vi "condAmbientalesFinales.vi"(8 "error in (no error)":errorcluster, 11 "Sonometro in":refnum<class "Sonometro.lvclass">) -> (0 "error out":errorcluster, 3 "Sonometro out":refnum<class "Sonometro.lvclass">)   [LabVIEW 2019, in "Sonometro.lvclass"]
uses:
  Sonometro.lvclass
  Base de Datos/Base de Datos.lvclass
  Base de Datos/SQLiteConnector/SQLiteConnection.lvclass
panel:
  in  "salir":bool
  in  "presion":dbl
  out "presion_corregida":dbl
  out "presion_ok":bool
  in  "humedad":dbl
  out "humedad_corregida":dbl
  out "humedad_ok":bool
  in  "temperatura":dbl
  out "temp_corregida":dbl
  out "temp_ok":bool
  # "Medido"
  # "Corregido"
  # "Cumple"
  # "Humedad [%]"
  # "Presión [hPa]"
  # "Temperatura [°C]"
  # "Condiciones Ambientales \nFINALES"
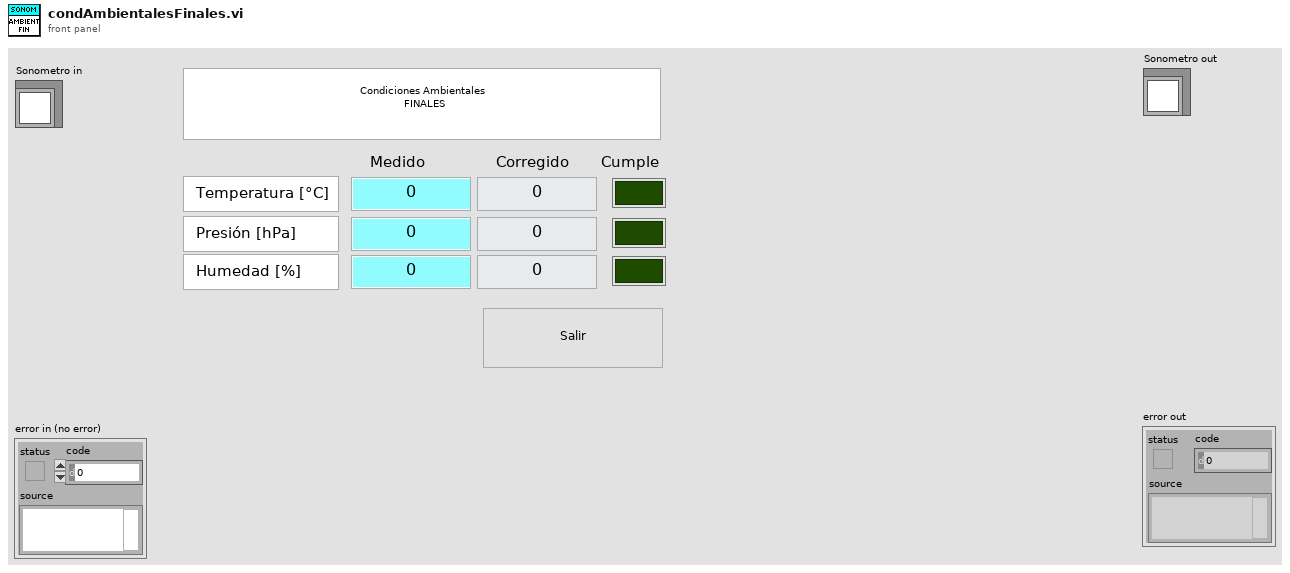
[diagram p1: front panel]
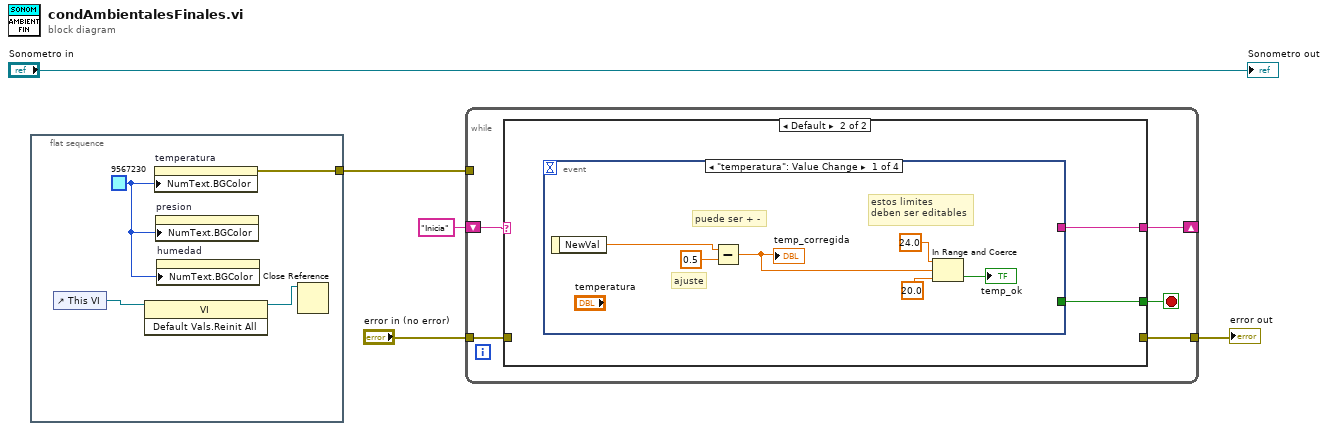
[diagram p0: block diagram]
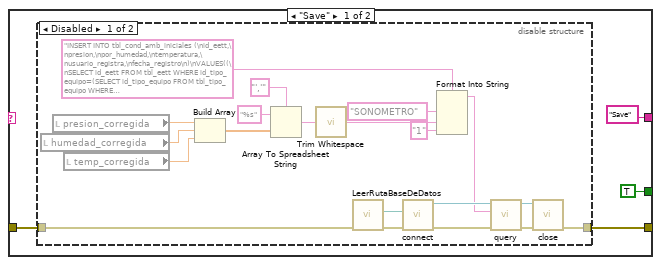
[diagram p2: hidden frame]
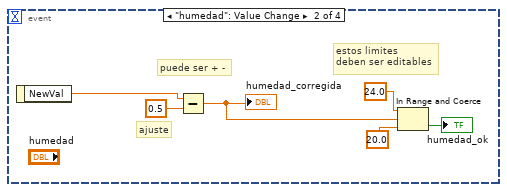
[diagram p4: hidden frame]
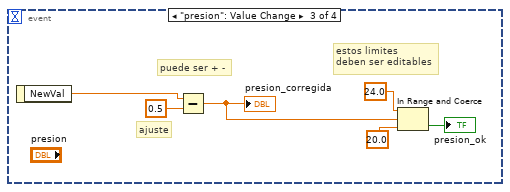
[diagram p5: hidden frame]
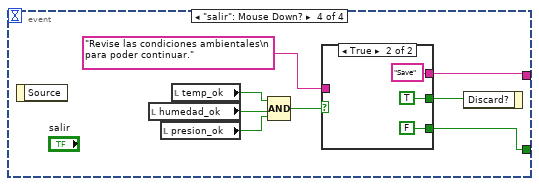
[diagram p6: hidden frame]
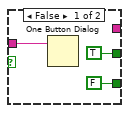
[diagram p7: hidden frame]
diagram:
  n1 = flat-sequence {
    tunnel: [w8] -> w4
    frame #0 {
      w9 = u32 9567230
      n2 = control-ref of="This VI"() -> (w7:refnum<vi>)
      n3 = invoke class="VI" method="Default Vals.Reinit All"(reference=w7) -> (reference out=w6:refnum<vi>)  [unwired: 2 in, 2 out]
      n4 = property on="temperatura" class="DigNum (strict)"("NumText.BGColor"=w9) -> (error out=w8:errorcluster)  [unwired: 2 in, 1 out]
      n5 = property on="presion" class="DigNum (strict)"("NumText.BGColor"=w9) -> ()  [unwired: 2 in, 2 out]
      n6 = property on="humedad" class="DigNum (strict)"("NumText.BGColor"=w9) -> ()  [unwired: 2 in, 2 out]
      n7 = Close Reference(reference=w6) -> ()  [unwired: 1 in, 1 out]
    }
  }
  n8 = while {
    tunnel: w4 -> [_]
    shift-right: [w12] -> _
    shift-left: "Inicia" -> [w13]
    tunnel: [w11] -> w1
    tunnel: "error in (no error)" -> [w10]
    stop <- w14 stop-if-true
    n9 = case shown="Default" w13 {
      tunnel: [TRUE w41] -> w14
      tunnel: ["Save" w40] -> w12
      tunnel: [w16 _] -> w11
      tunnel: w10 -> [w15 _]
      frame "Save" {
        n10 = disable-structure shown="Disabled" {
          disable-tunnel: [w20 w39] -> w16
          disable-tunnel: w15 -> [w19 w39]
          frame Disabled {
            n11 = local read "humedad_corregida"() -> (w29:dbl)
            n12 = local read "presion_corregida"() -> (w28:dbl)
            n13 = local read "temp_corregida"() -> (w30:dbl)
            n14 = Build Array(w28, w29, w30) -> (w27:dbl[])
            n15 = Array To Spreadsheet String(delimiter (Tab)="','", array=w27, 3:"%s" ("format string")) -> (spreadsheet string=w23:string)
            n16 = call <vilib>:"Trim Whitespace.vi"("string"=w23) -> ("trimmed string"=w22:string)  [unwired: 1 in]
            n17 = call "LeerRutaBaseDeDatos.vi"("error in (no error)"=w19) -> ("error out"=w33:errorcluster, "Database Path"=w34:path)  [unwired: 9 in]
            n18 = call "connect.vi"("error in (no error)"=w33, "Database Path"=w34) -> ("error out"=w36:errorcluster, "object out"=w35:refnum<class "SQLiteConnection.lvclass">)  [unwired: 8 in]
            n19 = Format Into String(format string="INSERT INTO tbl_cond_amb_iniciales (\nid_eett,\npresion,\npor_humedad,\ntemperatura,\nusuario_registra,\nfecha_registro\n)\nVALUES((\nSELECT id_eett FROM tbl_eett WHERE id_tipo_equipo=(SELECT id_tipo_equipo FROM tbl_tipo_equipo WHERE nombre='%s')),'%s','%s',DATETIME('NOW'))" ("SQL Statement"), "SONOMETRO" ("input 1"), w22, "1" ("input 2")) -> (resulting string=w31:string)  [unwired: 2 in, 1 out]
            n20 = call "query.vi"("error in (no error)"=w36, "SQL Statement"=w31, "object in"=w35) -> ("error out"=w38:errorcluster, "object out"=w37:refnum<class "SQLiteConnection.lvclass">)  [unwired: 5 in, 2 out]
            n21 = call-dynamic "close.vi"("error in (no error)"=w38, "object in"=w37) -> ("error out"=w20:errorcluster)  [unwired: 8 in, 1 out]
          }
          frame Enabled {
            # "Cambiar a codigo para BD de condiciones ambientales finales en Sonometro"
          }
        }
      }
      frame Default {
        n22 = event shown="[0] \"temperatura\": Value Change" {
          selector: _ -> [_ _ _ _]
          dyn-events: _ -> [_ _ _ _]
          timeout: _ -> [_ _ _ _]
          tunnel: [_ _ _ w61] -> w41
          tunnel: [_ _ _ w60] -> w40
          event "temperatura": Value Change {
            # "estos limites\ndeben ser editables"
            # "puede ser + -"
            # "ajuste"
            n23 = event-data() -> ("NewVal"=w42:dbl)  [unwired: 1 in]
            n24 = Subtract(x=w42, y=0.5) -> (x-y=w47:dbl)
            "temp_corregida" <- w47
            n25 = In Range and Coerce(upper limit=24.0, x=w47, lower limit=20.0) -> (In Range?=→"temp_ok":bool)  [unwired: 1 out]
          }
          event "humedad": Value Change {
            # "estos limites\ndeben ser editables"
            # "puede ser + -"
            # "ajuste"
            n26 = event-data() -> ("NewVal"=w50:dbl)  [unwired: 1 in]
            n27 = Subtract(x=w50, y=0.5) -> (x-y=w49:dbl)
            "humedad_corregida" <- w49
            n28 = In Range and Coerce(upper limit=24.0, x=w49, lower limit=20.0) -> (In Range?=→"humedad_ok":bool)  [unwired: 1 out]
          }
          event "presion": Value Change {
            # "estos limites\ndeben ser editables"
            # "puede ser + -"
            # "ajuste"
            n29 = event-data() -> ("NewVal"=w56:dbl)  [unwired: 1 in]
            n30 = Subtract(x=w56, y=0.5) -> (x-y=w55:dbl)
            "presion_corregida" <- w55
            n31 = In Range and Coerce(upper limit=24.0, x=w55, lower limit=20.0) -> (In Range?=→"presion_ok":bool)  [unwired: 1 out]
          }
          event "salir": Mouse Down? {
            n32 = event-data() -> ()  [unwired: 1 in, 1 out]
            n33 = local read "humedad_ok"() -> (w66:bool)
            n34 = local read "presion_ok"() -> (w65:bool)
            n35 = local read "temp_ok"() -> (w67:bool)
            n36 = Compound Arithmetic op=AND(w67, w66, w65) -> (w64:bool)
            n37 = case shown="True" w64 {
              tunnel: "Revise las condiciones ambientales\n           para poder continuar." -> [w70 _]
              tunnel: [TRUE TRUE] -> w62
              tunnel: [FALSE FALSE] -> w61
              tunnel: [_ "Save"] -> w60
              frame False {
                n38 = One Button Dialog(message=w70) -> ()  [unwired: 1 in, 1 out]
              }
              frame True {
              }
            }
            n39 = event-data("Discard?"=w62) -> ()  [unwired: 1 in, 1 out]
          }
        }
      }
    }
  }
  "error out" <- w1
  "Sonometro out" <- "Sonometro in"
